vi "niScope Acquisition Status.vi"(0 "instrument handle":refnum<k15>, 11 "error in":errorcluster) -> (4 "instrument handle out":refnum<k15>, 8 "acquisition status":i32, 15 "error out":errorcluster)   [LabVIEW 2011]
doc: "Returns status information indicating whether an acquisition is in progress, complete, or unknown to the <B>acquisition status</B> output parameter."
uses:
  niScope_32.dll
panel:
  # "Status Values:\n-1 = Status unknown\n0  = Acq. in progress\n1  = Acq. complete"
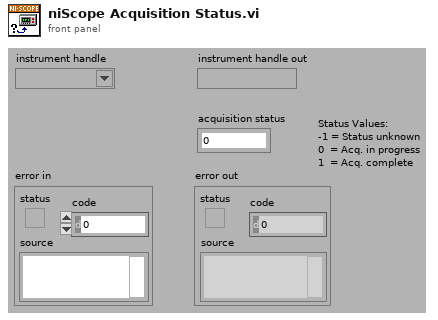
[diagram p1: front panel]
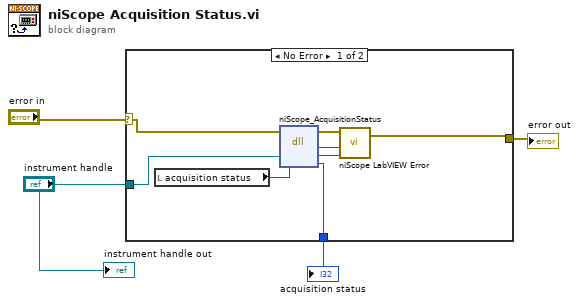
[diagram p0: block diagram]
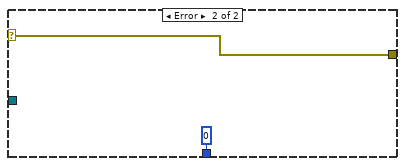
[diagram p2: hidden frame]
diagram:
  n1 = case shown="No Error" "error in" {
    selector: "error in" -> [w5 w12]
    tunnel: [w6 w12] -> w4
    tunnel: "instrument handle" -> [w11 _]
    tunnel: [w9 0 ("acquisition status")] -> w2
    frame No Error {
      n2 = local read "acquisition status"() -> (w10:i32)
      n3 = dll-call lib="niScope_*.*" fn="niScope_AcquisitionStatus"("instrument handle"=w11, "status"=w10) -> ("status"=w7:i32, "instrument handle"=w8:u32, "status"=w9:i32)  [unwired: 3 in, 2 out]
      n4 = call <instrlib>:"niScope LabVIEW Error.vi"("instrument handle"=w8, "niScope error code (0)"=w7, "error in (no error)"=w5) -> ("error out"=w6:errorcluster)  [unwired: 2 in]
    }
    frame Error {
    }
  }
  "error out" <- w4
  "acquisition status" <- w2
  "instrument handle out" <- "instrument handle"
